vi "ApplyMAXConfigurationFile.vi"(8 "error in (no error)":errorcluster, 11 "MAX Configuration File (*.nce)":path) -> (0 "error out":errorcluster)   [LabVIEW 2009]
uses:
  <userlib>/_OpenG.lib/file/file.llb/Strip Path Extension - String__ogtk.vi
panel:
  out "MAX Configuration Filename":string
  # "Applying Hardware Configuration"
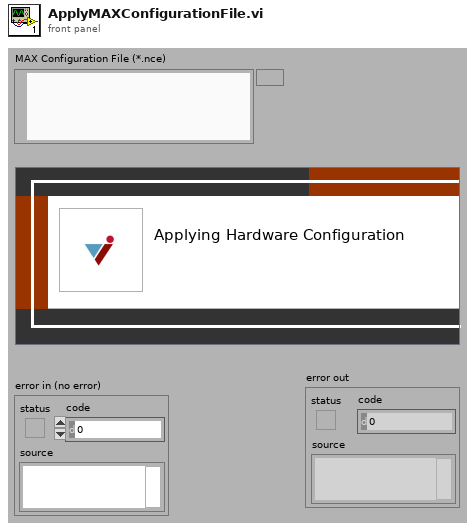
[diagram p1: front panel]
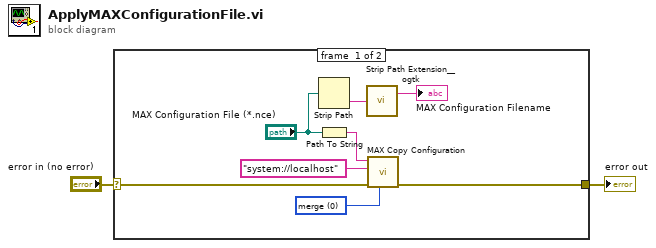
[diagram p0: block diagram]
diagram:
  n1 = case shown="No Error" "error in (no error)" {
    selector: "error in (no error)" -> [w6 w11]
    tunnel: [w7 w11] -> w1
    frame #0 {
      w10 = u32 0 items=["replace"=1048576, "merge"=0] ("replace mode")
      n2 = Strip Path(path="MAX Configuration File (*.nce)") -> (name=w4:string)  [unwired: 1 out]
      n3 = Path To String(path="MAX Configuration File (*.nce)") -> (string=w9:string)
      n4 = call-poly <userlib>:"Strip Path Extension__ogtk.vi"("path"=w4) -> ("root"=→"MAX Configuration Filename":string)  [unwired: 1 out]
      n5 = call <vilib>:"MAX Copy Configuration.vi"("replace mode"=w10, "error in (no error)"=w6, "destination"="system://localhost", "source"=w9) -> ("error out"=w7:errorcluster)  [unwired: 7 in]
    }
    frame #1 {
    }
  }
  "error out" <- w1
